vi "small current measurement.vi"() -> ()   [LabVIEW 2016]
doc: "This vi shows all current measurements in small format"
uses:
  Controls/Faraday cup states.ctl
panel:
  in  "Tab Control":enum32{"Measurements", "Errors"}(tab)
  out "cup being read":string
  out "Current measurements":dbl(graph)
  out "Current":dbl format="%#_4p"
  in  "stop":bool
  out "offset cup Actual":dbl format="%#_5g"
  out "VI error":errorcluster
  out "Beam Current":dbl format="%#_3p"
  out "rare count rate read error":errorcluster
  out "Inj current SV read error":errorcluster
  out "Keithley Error":errorcluster
  out "FC Status Read Error":errorcluster
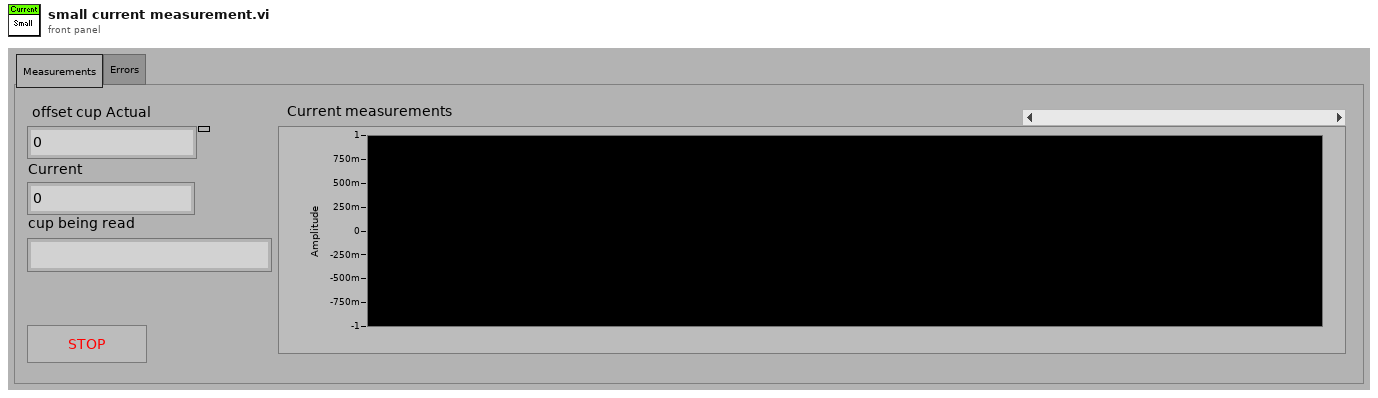
[diagram p1: front panel]
types:
  T1 = typedef "Faraday cup states.ctl" = enum16{"FC status unclear", "FC in", "FC out"}
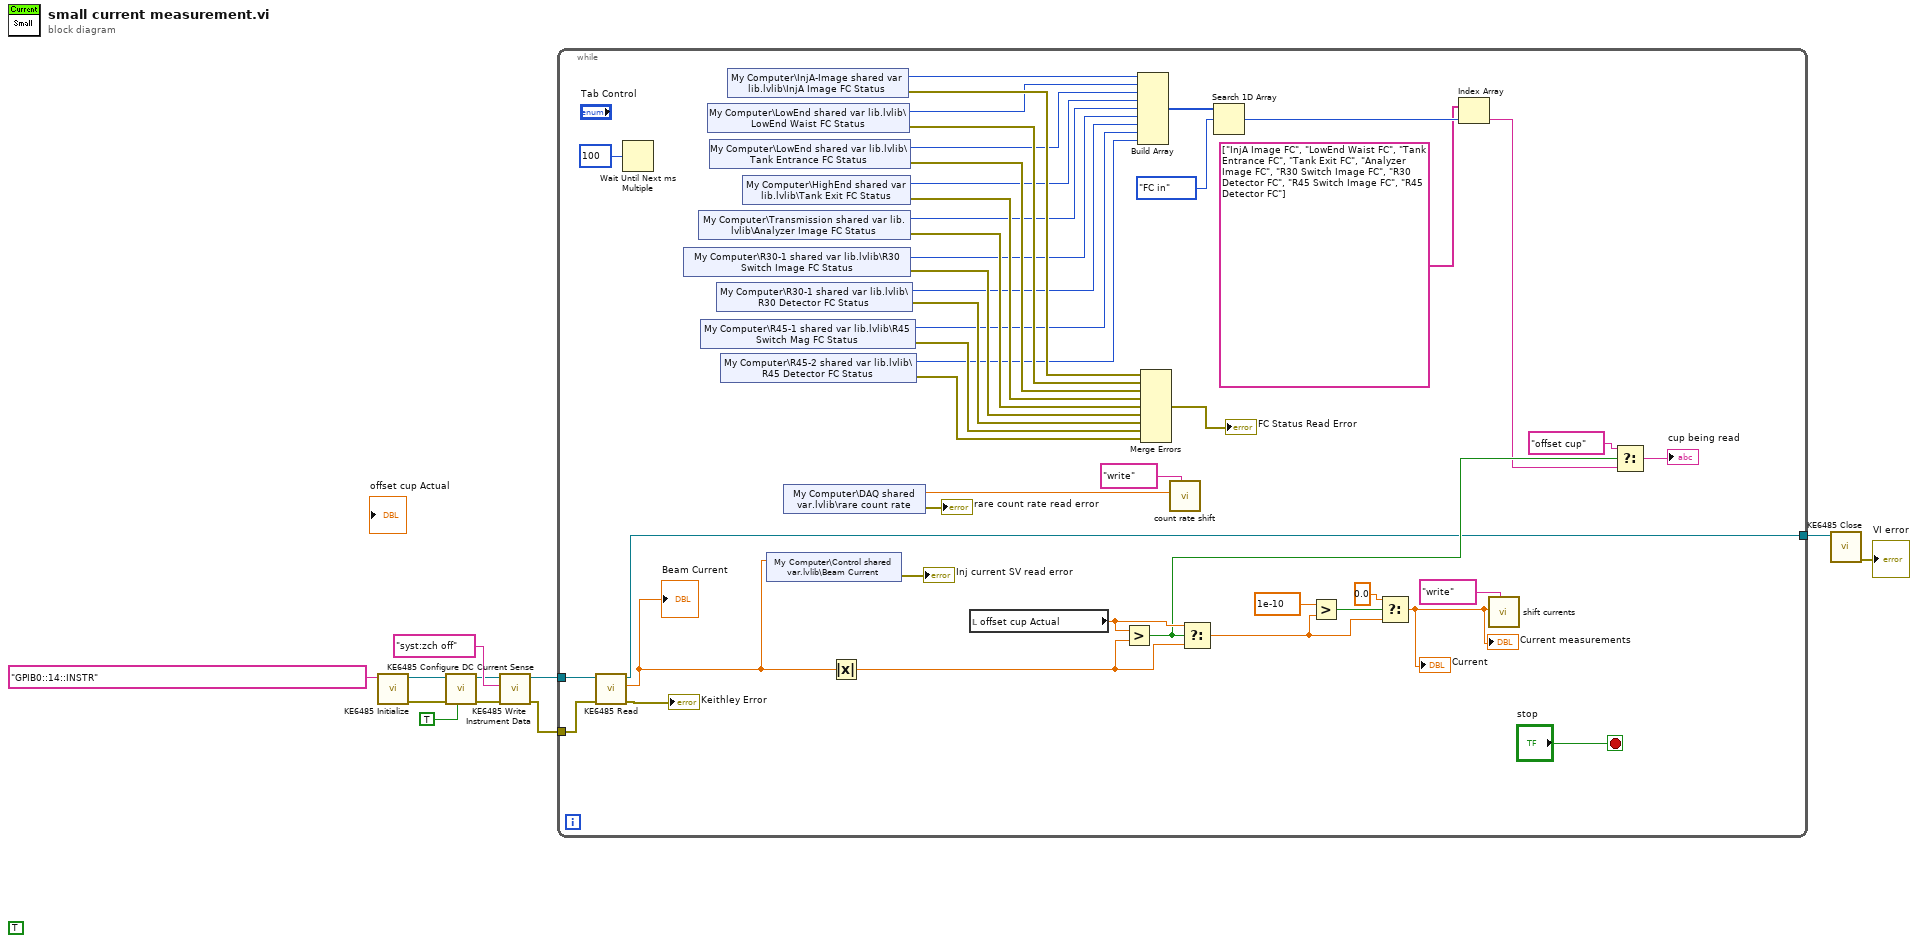
[diagram p0: block diagram]
diagram:
  (unwired) TRUE ("autorange")
  n1 = call "KE6485 Initialize.vi"("resource name"="GPIB0::14::INSTR") -> ("error out"=w8:errorcluster, "instrument handle out"=w7:refnum<k15>)  [unwired: 3 in, 6 out]
  n2 = call "KE6485 Configure DC Current Sense.vi"("autorange"=TRUE, "error in (no error)"=w8, "instrument handle"=w7) -> ("error out"=w10:errorcluster, "instrument handle out"=w9:refnum<k15>)  [unwired: 3 in, 4 out]
  n3 = call "KE6485 Write Instrument Data.vi"("error in (no error)"=w10, "write buffer"="syst:zch off" ("resource name"), "instrument handle"=w9) -> ("error out"=w4:errorcluster, "instrument handle out"=w5:refnum<k15>)  [unwired: 7 out]
  n4 = while {
    tunnel: w5 -> [w55]
    tunnel: w4 -> [w14]
    tunnel: [w39] -> w2
    stop <- "stop" stop-if-true
    n5 = call "KE6485 Read.vi"("error in (no error)"=w14, "instrument handle"=w55) -> ("error out"=→"Keithley Error":errorcluster, "reading"=w40:dbl, "instrument handle out"=w39:refnum<k15>)  [unwired: 1 in, 6 out]
    "Beam Current" <- w40
    n6 = Wait Until Next ms Multiple(millisecond multiple=u32 100) -> ()  [unwired: 1 out]
    n7 = shared-variable "My Computer\\R30-1 shared var lib.lvlib\\R30 Switch Image FC Status"() -> (w23:T1, error out=w32:errorcluster)  [unwired: 1 in]
    n8 = shared-variable "My Computer\\Transmission shared var lib.lvlib\\Analyzer Image FC Status"() -> (w24:T1, error out=w33:errorcluster)  [unwired: 1 in]
    n9 = shared-variable "My Computer\\R45-1 shared var lib.lvlib\\R45 Switch Mag FC Status"() -> (w21:T1, error out=w30:errorcluster)  [unwired: 1 in]
    n10 = shared-variable "My Computer\\LowEnd shared var lib.lvlib\\LowEnd Waist FC Status"() -> (w27:T1, error out=w36:errorcluster)  [unwired: 1 in]
    n11 = shared-variable "My Computer\\LowEnd shared var lib.lvlib\\Tank Entrance FC Status"() -> (w26:T1, error out=w35:errorcluster)  [unwired: 1 in]
    n12 = shared-variable "My Computer\\R30-1 shared var lib.lvlib\\R30 Detector FC Status"() -> (w22:T1, error out=w31:errorcluster)  [unwired: 1 in]
    n13 = shared-variable "My Computer\\R45-2 shared var lib.lvlib\\R45 Detector FC Status"() -> (w20:T1, error out=w29:errorcluster)  [unwired: 1 in]
    n14 = shared-variable "My Computer\\InjA-Image shared var lib.lvlib\\InjA Image FC Status"() -> (w28:T1, error out=w37:errorcluster)  [unwired: 1 in]
    n15 = shared-variable "My Computer\\HighEnd shared var lib.lvlib\\Tank Exit FC Status"() -> (w25:T1, error out=w34:errorcluster)  [unwired: 1 in]
    n16 = shared-variable "My Computer\\Control shared var.lvlib\\Beam Current"(w40) -> (error out=→"Inj current SV read error":errorcluster)  [unwired: 1 in]
    n17 = shared-variable "My Computer\\DAQ shared var.lvlib\\rare count rate"() -> (w43:dbl, error out=→"rare count rate read error":errorcluster)  [unwired: 1 in]
    n18 = Absolute Value(x=w40) -> (abs(x)=w38:dbl)
    n19 = local read "offset cup Actual"() -> (w49:dbl)
    n20 = Greater?(x=w49, y=w38) -> (0:w47:bool)
    n21 = Build Array(w28, w27, w26, w25, w24, w23, w22, w21, w20) -> (w19:T1[])
    n22 = Merge Errors(w37, w36, w35, w34, w33, w32, w31, w30, w29) -> (→"FC Status Read Error":errorcluster)
    n23 = call "count rate shift.vi"("read or write"="write" ("Combo Box"), "count rate in"=w43) -> ()  [unwired: 9 in, 1 out]
    n24 = Select(t=w49, s=w47, f=w38) -> (s? t:f=w48:dbl)
    n25 = Search 1D Array(1D array=w19, element=Faraday_cup_states."FC in") -> (index of element=w17:i32)  [unwired: 1 in]
    n26 = Greater?(x=1e-10, y=w48) -> (0:w53:bool)
    n27 = Select(t=0.0, s=w53, f=w48) -> (s? t:f=w50:dbl)
    "Current" <- w50
    "Current measurements" <- w50
    n28 = Index Array(array=string[] ["InjA Image FC", "LowEnd Waist FC", "Tank Entrance FC", "Tank Exit FC", "Analyzer Image FC", "R30 Switch Image FC", "R30 Detector FC", "R45 Switch Image FC", "R45 Detector FC"], index=w17) -> (element=w15:string)
    n29 = call "shift currents.vi"("Combo Box"="write", "current in"=w50) -> ()  [unwired: 9 in, 1 out]
    n30 = Select(t="offset cup", s=w47, f=w15) -> (s? t:f=→"cup being read":string)
  }
  n31 = call "KE6485 Close.vi"("instrument handle"=w2) -> ("error out"=→"VI error":errorcluster)  [unwired: 1 in, 9 out]
